vi "Start Triggers Time Core.vi"(0 "rx 1.stream enable":bool, 1 "rx.software trigger":bool, 2 "tx.trigger select":T4=enum."Immediate", 3 "tx.trigger enable":bool, 4 "tx 0.stream enable":bool, 5 "tx 1.stream enable":bool, 6 "rx 0.stream enable":bool, 7 "tx.software trigger":bool, 8 "rx.trigger enable":bool, 9 "time.resources":T3, 10 "rx.trigger select":T4=enum."Immediate") -> (14 "rx.start trigger":bool, 15 "tx.start trigger":bool)   [LabVIEW 2023]
uses:
  <instrlib>/niUSRPRIO/Time/v1/FPGA/niUsrpRio Time v1 FPGA.lvlib
  <instrlib>/niUSRP/Reference FPGA/USRPRIO Sample VIs/Host/SubVIs/Start Trigger.ctl
  <instrlib>/niUSRPRIO/Time/v1/FPGA/Private/Time Resources.ctl
  <instrlib>/niUSRPRIO/Time/v1/FPGA/Private/Future Event Resources.ctl
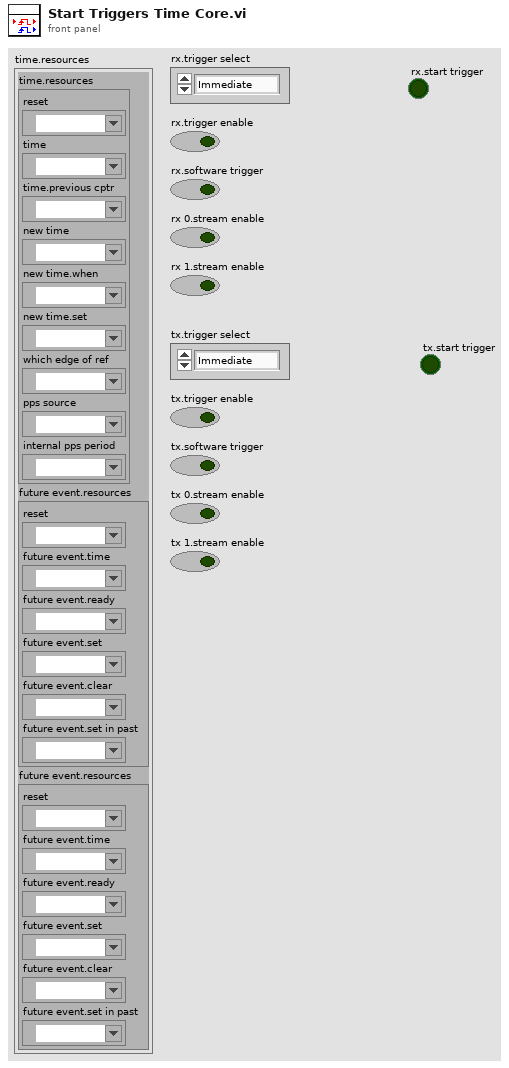
[diagram p1: front panel]
types:
  T1 = typedef "niUsrpRio Time v1 FPGA.lvlib/Time Resources.ctl" = cluster{"reset":refnum<k21>, "time":refnum<k21>, "time.previous cptr":refnum<k21>, "new time":refnum<k21>, "new time.when":refnum<k21>, "new time.set":refnum<k21>, "which edge of ref":refnum<k21>, "pps source":refnum<k21>, "internal pps period":refnum<k21>}
  T2 = typedef "niUsrpRio Time v1 FPGA.lvlib/Future Event Resources.ctl" = cluster{"reset":refnum<k21>, "future event.time":refnum<k21>, "future event.ready":refnum<k21>, "future event.set":refnum<k21>, "future event.clear":refnum<k21>, "future event.set in past":refnum<k21>}
  T3 = cluster{"time.resources":T1, "future event.resources":T2, "future event.resources":T2}
  T4 = typedef "Start Trigger.ctl" = enum8{"Software", "Digital Edge", "Rx Start Trigger", "Tx Start Trigger", "Immediate", "Future Time Event"}
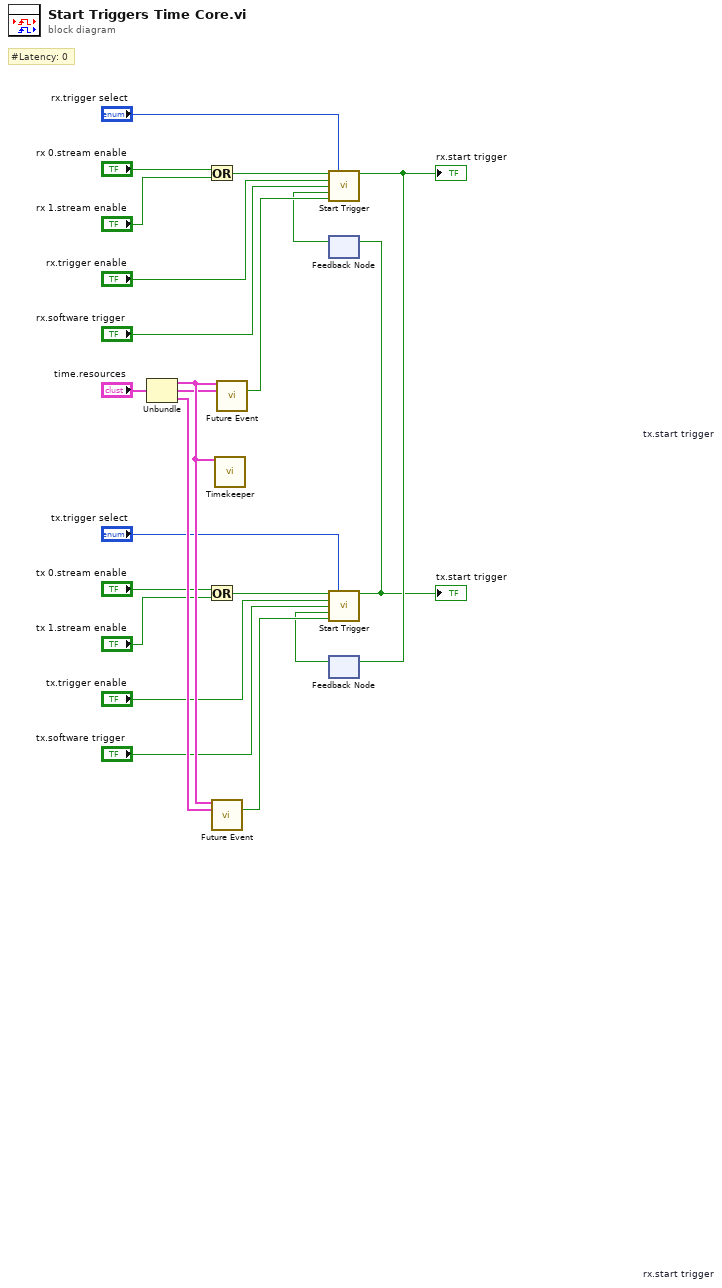
[diagram p0: block diagram]
diagram:
  # "#Latency: 0"
  n1 = Unbundle("time.resources") -> ("time.resources"=w22:T1, "future event.resources"=w1:T2, "future event.resources"=w21:T2)
  n2 = Or(x="rx 0.stream enable", y="rx 1.stream enable") -> (x .or. y?=w8:bool)
  n3 = Or(x="tx 0.stream enable", y="tx 1.stream enable") -> (x .or. y?=w7:bool)
  n4 = call <instrlib>:"Future Event.vi"("time.resources"=w22, "future event.resources"=w21) -> ("event.occurred"=w14:bool)  [unwired: 12 in, 1 out]
  n5 = call <instrlib>:"Timekeeper.vi"("time.resources"=w22) -> ()  [unwired: 13 in, 2 out]
  n6 = call <instrlib>:"Future Event.vi"("time.resources"=w22, "future event.resources"=w1) -> ("event.occurred"=w13:bool)  [unwired: 12 in, 1 out]
  n7 = feedback #1 "tx.start trigger"() -> (w3:bool)  [unwired: 1 in]
  n8 = call <instrlib>:"Start Trigger.vi"("stream enable"=w8, "trigger select"="rx.trigger select", "trigger enable"="rx.trigger enable", "software trigger"="rx.software trigger", "other start trigger"=w3, "event occurred"=w13) -> ("start trigger"=w16:bool)  [unwired: 9 in]
  "rx.start trigger" <- w16
  n9 = feedback-in #2(w16) -> ()
  n10 = feedback #2 "rx.start trigger"() -> (w4:bool)  [unwired: 1 in]
  n11 = call <instrlib>:"Start Trigger.vi"("stream enable"=w7, "trigger select"="tx.trigger select", "trigger enable"="tx.trigger enable", "software trigger"="tx.software trigger", "other start trigger"=w4, "event occurred"=w14) -> ("start trigger"=w15:bool)  [unwired: 9 in]
  "tx.start trigger" <- w15
  n12 = feedback-in #1(w15) -> ()
